vi "UI-Cmd-Quit.vi"(9 "Data":variant, 10 "Queue":refnum<queue>, 11 "UI State In":T1) -> (0 "error out":errorcluster, 3 "UI State Out":T1)   [LabVIEW 2024, in "CustomActions.lvlib"]
uses:
  CustomActions.lvlib
  UI-State--cluster.ctl
  UI-Refs--cluster.ctl
  UI-Platform--radio.ctl
  UI-ErrorCheckingLevel--radio.ctl
  UI-Cmd--cluster.ctl
  UI-Cmd--enum.ctl
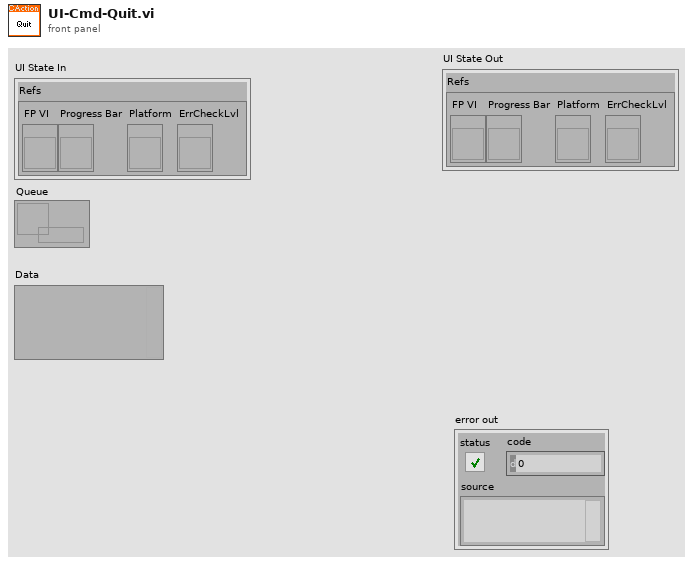
[diagram p1: front panel]
types:
  T1 = typedef "CustomActions.lvlib/UI-State--cluster.ctl" = cluster{"Refs":T2}
  T2 = typedef "CustomActions.lvlib/UI-Refs--cluster.ctl" = cluster{"FP VI":refnum<vi>, "Progress Bar":refnum<vi>, "Platform":refnum<vi>, "ErrCheckLvl":refnum<vi>}
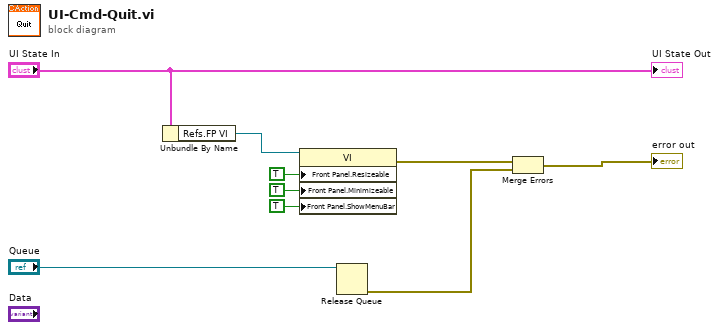
[diagram p0: block diagram]
diagram:
  n1 = Unbundle By Name("UI State In") -> ("Refs.FP VI"=w9:refnum<vi>)
  n2 = property class="VI"(reference=w9, "Front Panel.Resizeable"=TRUE ("Front Panel Window:Resizable"), "Front Panel.Minimizeable"=TRUE ("Front Panel Window:Minimizable"), "Front Panel.ShowMenuBar"=TRUE ("Front Panel Window:Show Menu Bar")) -> (error out=w4:errorcluster)  [unwired: 1 in, 1 out]
  n3 = Release Queue(queue="Queue") -> (error out=w1:errorcluster)  [unwired: 2 in, 2 out]
  n4 = Merge Errors(w4, w1) -> (→"error out":errorcluster)
  "UI State Out" <- "UI State In"
